vi "Get Producer Values.vi"(8 "error in":errorcluster, 11 "Climate Chamber Cluster.lvclass":refnum<class "Climate Chamber Cluster.lvclass">) -> (0 "error out":errorcluster, 1 "Producer Ch":T1(array[cluster]), 2 "Producer Control":T2, 3 "Climate Chamber Cluster.lvclass out":refnum<class "Climate Chamber Cluster.lvclass">)   [LabVIEW 2023, in "Climate Chamber Cluster.lvclass"]
uses:
  Climate Chamber Cluster.lvclass
  Climate Chamber Cluster.lvclass/Climate Chamber Cluster.ctl
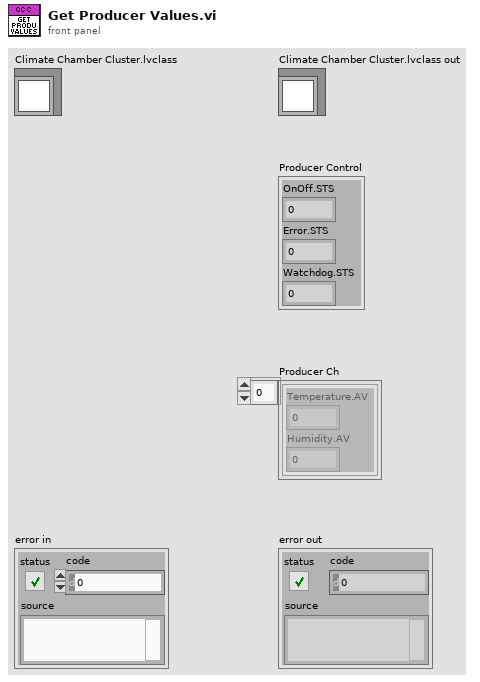
[diagram p1: front panel]
types:
  T1 = cluster{"Temperature.AV":dbl, "Humidity.AV":dbl}[]
  T2 = cluster{"OnOff.STS":i32, "Error.STS":i32, "Watchdog.STS":i32}
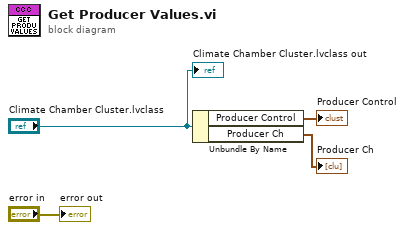
[diagram p0: block diagram]
diagram:
  n1 = Unbundle By Name("Climate Chamber Cluster.lvclass") -> ("Producer Control"=→"Producer Control":T2, "Producer Ch"=→"Producer Ch":T1)
  "error out" <- "error in"
  "Climate Chamber Cluster.lvclass out" <- "Climate Chamber Cluster.lvclass"
